vi "GeoData.vi"() -> ()   [LabVIEW 2017] (continued)
H1\n70391\t22007\tPaincourtville\tLA\tAssumption Parish\tH1\n70301\t22007\tThibodaux\tLA\tAssumption Parish\tH1\n70339\t22007\tPierre part\tLA\tAssumption Parish\tH1\n71362\t22009\tPlaucheville\tLA\tAvoyelles Parish\tH1\n71360\t22009\tPineville\tLA\tAvoyelles Parish\tH1\n71331\t22009\tEffie\tLA\tAvoyelles Parish\tH1\n71339\t22009\tHamburg\tLA\tAvoyelles Parish\tH1\n71350\t22009\tMansura\tLA\tAvoyelles Parish\tH1\n71353\t22009\tMelville\tLA\tAvoyelles Parish\tH1\n71355\t22009\tMoreauville\tLA\tAvoyelles Parish\tH1\n71328\t22009\tDeville\tLA\tAvoyelles Parish\tH1\n71323\t22009\tCenter point\tLA\tAvoyelles Parish\tH1\n71367\t22009\tSaint landry\tLA\tAvoyelles Parish\tH1\n71322\t22009\tBunkie\tLA\tAvoyelles Parish\tH1\n71327\t22009\tCottonport\tLA\tAvoyelles Parish\tH1\n71320\t22009\tBordelonville\tLA\tAvoyelles Parish\tH1\n71369\t22009\tSimmesport\tLA\tAvoyelles Parish\tH1\n71329\t22009\tDupont\tLA\tAvoyelles Parish\tH1\n71351\t22009\tMarksville\tLA\tAvoyelles Parish\tH1\n71341\t22009\tHessmer\tLA\tAvoyelles Parish\tH1\n71356\t22009\tMorrow\tLA\tAvoyelles Parish\tH1\n71333\t22009\tEvergreen\tLA\tAvoyelles Parish\tH1\n70653\t22011\tMerryville\tLA\tBeauregard Parish\tH1\n70662\t22011\tSugartown\tLA\tBeauregard Parish\tH1\n70633\t22011\tDequincy\tLA\tBeauregard Parish\tH1\n70637\t22011\tDry creek\tLA\tBeauregard Parish\tH1\n70634\t22011\tDeridder\tLA\tBeauregard Parish\tH1\n70657\t22011\tRagley\tLA\tBeauregard Parish\tH1\n70660\t22011\tSinger\tLA\tBeauregard Parish\tH1\n70652\t22011\tLongville\tLA\tBeauregard Parish\tH1\n70661\t22011\tStarks\tLA\tBeauregard Parish\tH1\n71070\t22013\tSaline\tLA\tBienville Parish\tH1\n71008\t22013\tBienville\tLA\tBienville Parish\tH1\n71275\t22013\tSimsboro\tLA\tBienville Parish\tH1\n71016\t22013\tCastor\tLA\tBienville Parish\tH1\n71024\t22013\tDubberly\tLA\tBienville Parish\tH1\n71055\t22013\tMinden\tLA\tBienville Parish\tH1\n71028\t22013\tGibsland\tLA\tBienville Parish\tH1\n71045\t22013\tJamestown\tLA\tBienville Parish\tH1\n71268\t22013\tQuitman\tLA\tBienville Parish\tH1\n71039\t22013\tHeflin\tLA\tBienville Parish\tH1\n71001\t22013\tArcadia\tLA\tBienville Parish\tH1\n71068\t22013\tRinggold\tLA\tBienville Parish\tH1\n71251\t22013\tJonesboro\tLA\tBienville Parish\tH1\n71080\t22013\tTaylor\tLA\tBienville Parish\tH1\n71006\t22015\tBenton\tLA\tBossier Parish\tH1\n71075\t22015\tSpringhill\tLA\tBossier Parish\tH1\n71067\t22015\tPrinceton\tLA\tBossier Parish\tH1\n71171\t22015\tBossier city\tLA\tBossier Parish\tH1\n71071\t22015\tSarepta\tLA\tBossier Parish\tH1\n71110\t22015\tBarksdale afb\tLA\tBossier Parish\tH1\n71111\t22015\tBossier city\tLA\tBossier Parish\tH1\n71105\t22015\tShreveport\tLA\tBossier Parish\tH1\n71113\t22015\tBossier city\tLA\tBossier Parish\tH1\n71106\t22015\tShreveport\tLA\tBossier Parish\tH1\n71104\t22015\tShreveport\tLA\tBossier Parish\tH1\n71101\t22015\tShreveport\tLA\tBossier Parish\tH1\n71137\t22015\tShreveport\tLA\tBossier Parish\tH1\n71112\t22015\tBossier city\tLA\tBossier Parish\tH1\n71172\t22015\tBossier city\tLA\tBossier Parish\tH1\n71064\t22015\tPlain dealing\tLA\tBossier Parish\tH1\n71115\t22015\tShreveport\tLA\tBossier Parish\tH1\n71051\t22015\tElm grove\tLA\tBossier Parish\tH1\n71037\t22015\tHaughton\tLA\tBossier Parish\tH1\n71023\t22015\tDoyline\tLA\tBossier Parish\tH1\n71107\t22015\tShreveport\tLA\tBossier Parish\tH1\n71018\t22015\tCotton valley\tLA\tBossier Parish\tH1\n71103\t22017\tShreveport\tLA\tCaddo Parish\tH1\n71004\t22017\tBelcher\tLA\tCaddo Parish\tH1\n71047\t22017\tKeithville\tLA\tCaddo Parish\tH1\n71046\t22017\tKeatchie\tLA\tCaddo Parish\tH1\n71044\t22017\tIda\tLA\tCaddo Parish\tH1\n71105\t22017\tShreveport\tLA\tCaddo Parish\tH1\n71134\t22017\tShreveport\tLA\tCaddo Parish\tH1\n71148\t22017\tShreveport\tLA\tCaddo Parish\tH1\n71029\t22017\tGilliam\tLA\tCaddo Parish\tH1\n71009\t22017\tBlanchard\tLA\tCaddo Parish\tH1\n71106\t22017\tShreveport\tLA\tCaddo Parish\tH1\n71104\t22017\tShreveport\tLA\tCaddo Parish\tH1\n71101\t22017\tShreveport\tLA\tCaddo Parish\tH1\n71061\t22017\tOil city\tLA\tCaddo Parish\tH1\n71136\t22017\tShreveport\tLA\tCaddo Parish\tH1\n71163\t22017\tShreveport\tLA\tCaddo Parish\tH1\n71109\t22017\tShreveport\tLA\tCaddo Parish\tH1\n71118\t22017\tShreveport\tLA\tCaddo Parish\tH1\n71119\t22017\tShreveport\tLA\tCaddo Parish\tH1\n71133\t22017\tShreveport\tLA\tCaddo Parish\tH1\n71033\t22017\tGreenwood\tLA\tCaddo Parish\tH1\n71060\t22017\tMooringsport\tLA\tCaddo Parish\tH1\n71069\t22017\tRodessa\tLA\tCaddo Parish\tH1\n71149\t22017\tShreveport\tLA\tCaddo Parish\tH1\n71162\t22017\tShreveport\tLA\tCaddo Parish\tH1\n71115\t22017\tShreveport\tLA\tCaddo Parish\tH1\n71043\t22017\tHosston\tLA\tCaddo Parish\tH1\n71165\t22017\tShreveport\tLA\tCaddo Parish\tH1\n71166\t22017\tShreveport\tLA\tCaddo Parish\tH1\n71129\t22017\tShreveport\tLA\tCaddo Parish\tH1\n71082\t22017\tVivian\tLA\tCaddo Parish\tH1\n71108\t22017\tShreveport\tLA\tCaddo Parish\tH1\n71138\t22017\tShreveport\tLA\tCaddo Parish\tH1\n71107\t22017\tShreveport\tLA\tCaddo Parish\tH1\n71135\t22017\tShreveport\tLA\tCaddo Parish\tH1\n71007\t22017\tBethany\tLA\tCaddo Parish\tH1\n71164\t22017\tShreveport\tLA\tCaddo Parish\tH1\n71161\t22017\tShreveport\tLA\tCaddo Parish\tH1\n71102\t22017\tShreveport\tLA\tCaddo Parish\tH1\n70605\t22019\tLake charles\tLA\tCalcasieu Parish\tH1\n70665\t22019\tSulphur\tLA\tCalcasieu Parish\tH1\n70601\t22019\tLake charles\tLA\tCalcasieu Parish\tH1\n70630\t22019\tBell city\tLA\tCalcasieu Parish\tH1\n70606\t22019\tLake charles\tLA\tCalcasieu Parish\tH1\n70633\t22019\tDequincy\tLA\tCalcasieu Parish\tH1\n70663\t22019\tSulphur\tLA\tCalcasieu Parish\tH1\n70612\t22019\tLake charles\tLA\tCalcasieu Parish\tH1\n70607\t22019\tLake charles\tLA\tCalcasieu Parish\tH1\n70629\t22019\tLake charles\tLA\tCalcasieu Parish\tH1\n70602\t22019\tLake charles\tLA\tCalcasieu Parish\tH1\n70647\t22019\tIowa\tLA\tCalcasieu Parish\tH1\n70657\t22019\tRagley\tLA\tCalcasieu Parish\tH1\n70646\t22019\tHayes\tLA\tCalcasieu Parish\tH1\n70611\t22019\tLake charles\tLA\tCalcasieu Parish\tH1\n70615\t22019\tLake charles\tLA\tCalcasieu Parish\tH1\n70669\t22019\tWestlake\tLA\tCalcasieu Parish\tH1\n70668\t22019\tVinton\tLA\tCalcasieu Parish\tH1\n70661\t22019\tStarks\tLA\tCalcasieu Parish\tH1\n70616\t22019\tLake charles\tLA\tCalcasieu Parish\tH1\n71465\t22021\tOlla\tLA\tCaldwell Parish\tH1\n71435\t22021\tGrayson\tLA\tCaldwell Parish\tH1\n71418\t22021\tColumbia\tLA\tCaldwell Parish\tH1\n71441\t22021\tKelly\tLA\tCaldwell Parish\tH1\n71415\t22021\tClarks\tLA\tCaldwell Parish\tH1\n70630\t22023\tBell city\tLA\tCameron Parish\tH1\n70542\t22023\tGueydan\tLA\tCameron Parish\tH1\n70645\t22023\tHackberry\tLA\tCameron Parish\tH1\n70606\t22023\tLake charles\tLA\tCameron Parish\tH1\n70643\t22023\tGrand chenier\tLA\tCameron Parish\tH1\n70607\t22023\tLake charles\tLA\tCameron Parish\tH1\n70631\t22023\tCameron\tLA\tCameron Parish\tH1\n70549\t22023\tLake arthur\tLA\tCameron Parish\tH1\n70632\t22023\tCreole\tLA\tCameron Parish\tH1\n71340\t22025\tHarrisonburg\tLA\tCatahoula Parish\tH1\n71363\t22025\tRhinehart\tLA\tCatahoula Parish\tH1\n71368\t22025\tSicily island\tLA\tCatahoula Parish\tH1\n71465\t22025\tOlla\tLA\tCatahoula Parish\tH1\n71354\t22025\tMonterey\tLA\tCatahoula Parish\tH1\n71401\t22025\tAimwell\tLA\tCatahoula Parish\tH1\n71418\t22025\tColumbia\tLA\tCatahoula Parish\tH1\n71425\t22025\tEnterprise\tLA\tCatahoula Parish\tH1\n71343\t22025\tJonesville\tLA\tCatahoula Parish\tH1\n71326\t22025\tClayton\tLA\tCatahoula Parish\tH1\n71256\t22027\tLillie\tLA\tClaiborne Parish\tH1\n71038\t22027\tHaynesville\tLA\tClaiborne Parish\tH1\n71048\t22027\tLisbon\tLA\tClaiborne Parish\tH1\n71222\t22027\tBernice\tLA\tClaiborne Parish\tH1\n71003\t22027\tAthens\tLA\tClaiborne Parish\tH1\n71055\t22027\tMinden\tLA\tClaiborne Parish\tH1\n71028\t22027\tGibsland\tLA\tClaiborne Parish\tH1\n71235\t22027\tDubach\tLA\tClaiborne Parish\tH1\n71001\t22027\tArcadia\tLA\tClaiborne Parish\tH1\n71040\t22027\tHomer\tLA\tClaiborne Parish\tH1\n71079\t22027\tSummerfield\tLA\tClaiborne Parish\tH1\n71373\t22029\tVidalia\tLA\tConcordia Parish\tH1\n71316\t22029\tAcme\tLA\tConcordia Parish\tH1\n71354\t22029\tMonterey\tLA\tConcordia Parish\tH1\n71334\t22029\tFerriday\tLA\tConcordia Parish\tH1\n71343\t22029\tJonesville\tLA\tConcordia Parish\tH1\n71326\t22029\tClayton\tLA\tConcordia Parish\tH1\n71063\t22031\tPelican\tLA\tDe Soto Parish\tH1\n71046\t22031\tKeatchie\tLA\tDe Soto Parish\tH1\n71030\t22031\tGloster\tLA\tDe Soto Parish\tH1\n71049\t22031\tLogansport\tLA\tDe Soto Parish\tH1\n71052\t22031\tMansfield\tLA\tDe Soto Parish\tH1\n71032\t22031\tGrand cane\tLA\tDe Soto Parish\tH1\n71078\t22031\tStonewall\tLA\tDe Soto Parish\tH1\n71419\t22031\tConverse\tLA\tDe Soto Parish\tH1\n71027\t22031\tFrierson\tLA\tDe Soto Parish\tH1\n70805\t22033\tBaton rouge\tLA\tEast Baton Rouge Parish\tH1\n70815\t22033\tBaton rouge\tLA\tEast Baton Rouge Parish\tH1\n70770\t22033\tPride\tLA\tEast Baton Rouge Parish\tH1\n70802\t22033\tBaton rouge\tLA\tEast Baton Rouge Parish\tH1\n70814\t22033\tBaton rouge\tLA\tEast Baton Rouge Parish\tH1\n70817\t22033\tBaton rouge\tLA\tEast Baton Rouge Parish\tH1\n70898\t22033\tBaton rouge\tLA\tEast Baton Rouge Parish\tH1\n70819\t22033\tBaton rouge\tLA\tEast Baton Rouge Parish\tH1\n70827\t22033\tBaton rouge\tLA\tEast Baton Rouge Parish\tH1\n70810\t22033\tBaton rouge\tLA\tEast Baton Rouge Parish\tH1\n70748\t22033\tJackson\tLA\tEast Baton Rouge Parish\tH1\n70812\t22033\tBaton rouge\tLA\tEast Baton Rouge Parish\tH1\n70835\t22033\tBaton rouge\tLA\tEast Baton Rouge Parish\tH1\n70879\t22033\tBaton rouge\tLA\tEast Baton Rouge Parish\tH1\n70777\t22033\tSlaughter\tLA\tEast Baton Rouge Parish\tH1\n70807\t22033\tBaton rouge\tLA\tEast Baton Rouge Parish\tH1\n70739\t22033\tGreenwell springs\tLA\tEast Baton Rouge Parish\tH1\n70804\t22033\tBaton rouge\tLA\tEast Baton Rouge Parish\tH1\n70874\t22033\tBaton rouge\tLA\tEast Baton Rouge Parish\tH1\n70896\t22033\tBaton rouge\tLA\tEast Baton Rouge Parish\tH1\n70722\t22033\tClinton\tLA\tEast Baton Rouge Parish\tH1\n70806\t22033\tBaton rouge\tLA\tEast Baton Rouge Parish\tH1\n70808\t22033\tBaton rouge\tLA\tEast Baton Rouge Parish\tH1\n70821\t22033\tBaton rouge\tLA\tEast Baton Rouge Parish\tH1\n70714\t22033\tBaker\tLA\tEast Baton Rouge Parish\tH1\n70818\t22033\tBaton rouge\tLA\tEast Baton Rouge Parish\tH1\n70836\t22033\tBaton rouge\tLA\tEast Baton Rouge Parish\tH1\n70892\t22033\tBaton rouge\tLA\tEast Baton Rouge Parish\tH1\n70884\t22033\tBaton rouge\tLA\tEast Baton Rouge Parish\tH1\n70893\t22033\tBaton rouge\tLA\tEast Baton Rouge Parish\tH1\n70809\t22033\tBaton rouge\tLA\tEast Baton Rouge Parish\tH1\n70801\t22033\tBaton rouge\tLA\tEast Baton Rouge Parish\tH1\n70791\t22033\tZachary\tLA\tEast Baton Rouge Parish\tH1\n70811\t22033\tBaton rouge\tLA\tEast Baton Rouge Parish\tH1\n70767\t22033\tPort allen\tLA\tEast Baton Rouge Parish\tH1\n70816\t22033\tBaton rouge\tLA\tEast Baton Rouge Parish\tH1\n70820\t22033\tBaton rouge\tLA\tEast Baton Rouge Parish\tH1\n70825\t22033\tBaton rouge\tLA\tEast Baton Rouge Parish\tH1\n70895\t22033\tBaton rouge\tLA\tEast Baton Rouge Parish\tH1\n70704\t22033\tBaker\tLA\tEast Baton Rouge Parish\tH1\n70803\t22033\tBaton rouge\tLA\tEast Baton Rouge Parish\tH1\n71254\t22035\tLake providence\tLA\tEast Carroll Parish\tH1\n71286\t22035\tTransylvania\tLA\tEast Carroll Parish\tH1\n71276\t22035\tSondheimer\tLA\tEast Carroll Parish\tH1\n71237\t22035\tEpps\tLA\tEast Carroll Parish\tH1\n70748\t22037\tJackson\tLA\tEast Feliciana Parish\tH1\n70761\t22037\tNorwood\tLA\tEast Feliciana Parish\tH1\n70777\t22037\tSlaughter\tLA\tEast Feliciana Parish\tH1\n70722\t22037\tClinton\tLA\tEast Feliciana Parish\tH1\n70730\t22037\tEthel\tLA\tEast Feliciana Parish\tH1\n70791\t22037\tZachary\tLA\tEast Feliciana Parish\tH1\n70789\t22037\tWilson\tLA\tEast Feliciana Parish\tH1\n70580\t22039\tReddell\tLA\tEvangeline Parish\tH1\n70585\t22039\tTurkey creek\tLA\tEvangeline Parish\tH1\n70524\t22039\tChataignier\tLA\tEvangeline Parish\tH1\n70576\t22039\tPine prairie\tLA\tEvangeline Parish\tH1\n70586\t22039\tVille platte\tLA\tEvangeline Parish\tH1\n70589\t22039\tWashington\tLA\tEvangeline Parish\tH1\n71367\t22039\tSaint landry\tLA\tEvangeline Parish\tH1\n70554\t22039\tMamou\tLA\tEvangeline Parish\tH1\n70535\t22039\tEunice\tLA\tEvangeline Parish\tH1\n70515\t22039\tBasile\tLA\tEvangeline Parish\tH1\n71463\t22039\tOakdale\tLA\tEvangeline Parish\tH1\n71433\t22039\tGlenmora\tLA\tEvangeline Parish\tH1\n71325\t22039\tCheneyville\tLA\tEvangeline Parish\tH1\n70570\t22039\tOpelousas\tLA\tEvangeline Parish\tH1\n71269\t22041\tRayville\tLA\tFranklin Parish\tH1\n71368\t22041\tSicily island\tLA\tFranklin Parish\tH1\n71219\t22041\tBaskin\tLA\tFranklin Parish\tH1\n71243\t22041\tFort necessity\tLA\tFranklin Parish\tH1\n71295\t22041\tWinnsboro\tLA\tFranklin Parish\tH1\n71249\t22041\tJigger\tLA\tFranklin Parish\tH1\n71336\t22041\tGilbert\tLA\tFranklin Parish\tH1\n71378\t22041\tWisner\tLA\tFranklin Parish\tH1\n71230\t22041\tCrowville\tLA\tFranklin Parish\tH1\n71232\t22041\tDelhi\tLA\tFranklin Parish\tH1\n71324\t22041\tChase\tLA\tFranklin Parish\tH1\n71360\t22043\tPineville\tLA\tGrant Parish\tH1\n71407\t22043\tBentley\tLA\tGrant Parish\tH1\n71423\t22043\tDry prong\tLA\tGrant Parish\tH1\n71404\t22043\tAtlanta\tLA\tGrant Parish\tH1\n71454\t22043\tMontgomery\tLA\tGrant Parish\tH1\n71417\t22043\tColfax\tLA\tGrant Parish\tH1\n71432\t22043\tGeorgetown\tLA\tGrant Parish\tH1\n71467\t22043\tPollock\tLA\tGrant Parish\tH1\n70560\t22045\tNew iberia\tLA\tIberia Parish\tH1\n70592\t22045\tYoungsville\tLA\tIberia Parish\tH1\n70513\t22045\tAvery island\tLA\tIberia Parish\tH1\n70563\t22045\tNew iberia\tLA\tIberia Parish\tH1\n70569\t22045\tLydia\tLA\tIberia Parish\tH1\n70544\t22045\tJeanerette\tLA\tIberia Parish\tH1\n70533\t22045\tErath\tLA\tIberia Parish\tH1\n70528\t22045\tDelcambre\tLA\tIberia Parish\tH1\n70582\t22045\tSaint martinville\tLA\tIberia Parish\tH1\n70552\t22045\tLoreauville\tLA\tIberia Parish\tH1\n70562\t22045\tNew iberia\tLA\tIberia Parish\tH1\n70518\t22045\tBroussard\tLA\tIberia Parish\tH1\n70346\t22047\tDonaldsonville\tLA\tIberville Parish\tH1\n70764\t22047\tPlaquemine\tLA\tIberville Parish\tH1\n70740\t22047\tGrosse tete\tLA\tIberville Parish\tH1\n70721\t22047\tCarville\tLA\tIberville Parish\tH1\n70772\t22047\tRosedale\tLA\tIberville Parish\tH1\n70776\t22047\tSaint gabriel\tLA\tIberville Parish\tH1\n70757\t22047\tMaringouin\tLA\tIberville Parish\tH1\n70780\t22047\tSunshine\tLA\tIberville Parish\tH1\n70788\t22047\tWhite castle\tLA\tIberville Parish\tH1\n71238\t22049\tEros\tLA\tJackson Parish\tH1\n71435\t22049\tGrayson\tLA\tJackson Parish\tH1\n71225\t22049\tCalhoun\tLA\tJackson Parish\tH1\n71247\t22049\tHodge\tLA\tJackson Parish\tH1\n71268\t22049\tQuitman\tLA\tJackson Parish\tH1\n71226\t22049\tChatham\tLA\tJackson Parish\tH1\n71251\t22049\tJonesboro\tLA\tJackson Parish\tH1\n71227\t22049\tChoudrant\tLA\tJackson Parish\tH1\n71270\t22049\tRuston\tLA\tJackson Parish\tH1\n70058\t22051\tHarvey\tLA\tJefferson Parish\tH1\n70094\t22051\tWestwego\tLA\tJefferson Parish\tH1\n70064\t22051\tKenner\tLA\tJefferson Parish\tH1\n70073\t22051\tMarrero\tLA\tJefferson Parish\tH1\n70121\t22051\tNew orleans\tLA\tJefferson Parish\tH1\n70063\t22051\tKenner\tLA\tJefferson Parish\tH1\n70181\t22051\tNew orleans\tLA\tJefferson Parish\tH1\n70010\t22051\tMetairie\tLA\tJefferson Parish\tH1\n70003\t22051\tMetairie\tLA\tJefferson Parish\tH1\n70115\t22051\tNew orleans\tLA\tJefferson Parish\tH1\n70183\t22051\tNew orleans\tLA\tJefferson Parish\tH1\n70009\t22051\tMetairie\tLA\tJefferson Parish\tH1\n70055\t22051\tMetairie\tLA\tJefferson Parish\tH1\n70065\t22051\tKenner\tLA\tJefferson Parish\tH1\n70062\t22051\tKenner\tLA\tJefferson Parish\tH1\n70123\t22051\tNew orleans\tLA\tJefferson Parish\tH1\n70011\t22051\tMetairie\tLA\tJefferson Parish\tH1\n70005\t22051\tMetairie\tLA\tJefferson Parish\tH1\n70033\t22051\tMetairie\tLA\tJefferson Parish\tH1\n70031\t22051\tAma\tLA\tJefferson Parish\tH1\n70002\t22051\tMetairie\tLA\tJefferson Parish\tH1\n70053\t22051\tGretna\tLA\tJefferson Parish\tH1\n70067\t22051\tLafitte\tLA\tJefferson Parish\tH1\n70059\t22051\tHarvey\tLA\tJefferson Parish\tH1\n70006\t22051\tMetairie\tLA\tJefferson Parish\tH1\n70036\t22051\tBarataria\tLA\tJefferson Parish\tH1\n70004\t22051\tMetairie\tLA\tJefferson Parish\tH1\n70056\t22051\tGretna\tLA\tJefferson Parish\tH1\n70114\t22051\tNew orleans\tLA\tJefferson Parish\tH1\n70001\t22051\tMetairie\tLA\tJefferson Parish\tH1\n70054\t22051\tGretna\tLA\tJefferson Parish\tH1\n70072\t22051\tMarrero\tLA\tJefferson Parish\tH1\n70358\t22051\tGrand isle\tLA\tJefferson Parish\tH1\n70096\t22051\tWestwego\tLA\tJefferson Parish\tH1\n70591\t22053\tWelsh\tLA\tJefferson Davis Parish\tH1\n70640\t22053\tFenton\tLA\tJefferson Davis Parish\tH1\n70546\t22053\tJennings\tLA\tJefferson Davis Parish\tH1\n70650\t22053\tLacassine\tLA\tJefferson Davis Parish\tH1\n70549\t22053\tLake arthur\tLA\tJefferson Davis Parish\tH1\n70647\t22053\tIowa\tLA\tJefferson Davis Parish\tH1\n70532\t22053\tElton\tLA\tJefferson Davis Parish\tH1\n70657\t22053\tRagley\tLA\tJefferson Davis Parish\tH1\n70611\t22053\tLake charles\tLA\tJefferson Davis Parish\tH1\n70648\t22053\tKinder\tLA\tJefferson Davis Parish\tH1\n70581\t22053\tRoanoke\tLA\tJefferson Davis Parish\tH1\n70517\t22055\tBreaux bridge\tLA\tLafayette Parish\tH1\n70560\t22055\tNew iberia\tLA\tLafayette Parish\tH1\n70501\t22055\tLafayette\tLA\tLafayette Parish\tH1\n70506\t22055\tLafayette\tLA\tLafayette Parish\tH1\n70592\t22055\tYoungsville\tLA\tLafayette Parish\tH1\n70502\t22055\tLafayette\tLA\tLafayette Parish\tH1\n70503\t22055\tLafayette\tLA\tLafayette Parish\tH1\n70525\t22055\tChurch point\tLA\tLafayette Parish\tH1\n70558\t22055\tMilton\tLA\tLafayette Parish\tH1\n70507\t22055\tLafayette\tLA\tLafayette Parish\tH1\n70555\t22055\tMaurice\tLA\tLafayette Parish\tH1\n70508\t22055\tLafayette\tLA\tLafayette Parish\tH1\n70505\t22055\tLafayette\tLA\tLafayette Parish\tH1\n70578\t22055\tRayne\tLA\tLafayette Parish\tH1\n70529\t22055\tDuson\tLA\tLafayette Parish\tH1\n70504\t22055\tLafayette\tLA\tLafayette Parish\tH1\n70518\t22055\tBroussard\tLA\tLafayette Parish\tH1\n70520\t22055\tCarencro\tLA\tLafayette Parish\tH1\n70583\t22055\tScott\tLA\tLafayette Parish\tH1\n70596\t22055\tLafayette\tLA\tLafayette Parish\tH1\n70509\t22055\tLafayette\tLA\tLafayette Parish\tH1\n70598\t22055\tLafayette\tLA\tLafayette Parish\tH1\n70374\t22057\tLockport\tLA\tLafourche Parish\tH1\n70357\t22057\tGolden meadow\tLA\tLafourche Parish\tH1\n70343\t22057\tBourg\tLA\tLafourche Parish\tH1\n70354\t22057\tGalliano\tLA\tLafourche Parish\tH1\n70364\t22057\tHouma\tLA\tLafourche Parish\tH1\n70345\t22057\tCut off\tLA\tLafourche Parish\tH1\n70394\t22057\tRaceland\tLA\tLafourche Parish\tH1\n70355\t22057\tGheens\tLA\tLafourche Parish\tH1\n70359\t22057\tGray\tLA\tLafourche Parish\tH1\n70371\t22057\tKraemer\tLA\tLafourche Parish\tH1\n70301\t22057\tThibodaux\tLA\tLafourche Parish\tH1\n70375\t22057\tMathews\tLA\tLafourche Parish\tH1\n70030\t22057\tDes allemands\tLA\tLafourche Parish\tH1\n70377\t22057\tMontegut\tLA\tLafourche Parish\tH1\n70373\t22057\tLarose\tLA\tLafourche Parish\tH1\n71479\t22059\tTullos\tLA\tLa Salle Parish\tH1\n71465\t22059\tOlla\tLA\tLa Salle Parish\tH1\n71435\t22059\tGrayson\tLA\tLa Salle Parish\tH1\n71480\t22059\tUrania\tLA\tLa Salle Parish\tH1\n71441\t22059\tKelly\tLA\tLa Salle Parish\tH1\n71342\t22059\tJena\tLA\tLa Salle Parish\tH1\n71343\t22059\tJonesville\tLA\tLa Salle Parish\tH1\n71371\t22059\tTrout\tLA\tLa Salle Parish\tH1\n71275\t22061\tSimsboro\tLA\tLincoln Parish\tH1\n71272\t22061\tRuston\tLA\tLincoln Parish\tH1\n71234\t22061\tDownsville\tLA\tLincoln Parish\tH1\n71003\t22061\tAthens\tLA\tLincoln Parish\tH1\n71273\t22061\tRuston\tLA\tLincoln Parish\tH1\n71241\t22061\tFarmerville\tLA\tLincoln Parish\tH1\n71235\t22061\tDubach\tLA\tLincoln Parish\tH1\n71001\t22061\tArcadia\tLA\tLincoln Parish\tH1\n71227\t22061\tChoudrant\tLA\tLincoln Parish\tH1\n71245\t22061\tGrambling\tLA\tLincoln Parish\tH1\n71270\t22061\tRuston\tLA\tLincoln Parish\tH1\n70706\t22063\tDenham springs\tLA\tLivingston Parish\tH1\n70403\t22063\tHammond\tLA\tLivingston Parish\tH1\n70466\t22063\tTickfaw\tLA\tLivingston Parish\tH1\n70754\t22063\tLivingston\tLA\tLivingston Parish\tH1\n70774\t22063\tSaint amant\tLA\tLivingston Parish\tH1\n70727\t22063\tDenham springs\tLA\tLivingston Parish\tH1\n70726\t22063\tDenham springs\tLA\tLivingston Parish\tH1\n70711\t22063\tAlbany\tLA\tLivingston Parish\tH1\n70786\t22063\tWatson\tLA\tLivingston Parish\tH1\n70462\t22063\tSpringfield\tLA\tLivingston Parish\tH1\n70453\t22063\tPine grove\tLA\tLivingston Parish\tH1\n70449\t22063\tMaurepas\tLA\tLivingston Parish\tH1\n70422\t22063\tAmite\tLA\tLivingston Parish\tH1\n70443\t22063\tIndependence\tLA\tLivingston Parish\tH1\n70785\t22063\tWalker\tLA\tLivingston Parish\tH1\n70744\t22063\tHolden\tLA\tLivingston Parish\tH1\n70733\t22063\tFrench settlement\tLA\tLivingston Parish\tH1\n71233\t22065\tDelta\tLA\tMadison Parish\tH1\n71237\t22065\tEpps\tLA\tMadison Parish\tH1\n71232\t22065\tDelhi\tLA\tMadison Parish\tH1\n71282\t22065\tTallulah\tLA\tMadison Parish\tH1\n71280\t22067\tSterlington\tLA\tMorehouse Parish\tH1\n71261\t22067\tMer rouge\tLA\tMorehouse Parish\tH1\n71269\t22067\tRayville\tLA\tMorehouse Parish\tH1\n71223\t22067\tBonita\tLA\tMorehouse Parish\tH1\n71264\t22067\tOak ridge\tLA\tMorehouse Parish\tH1\n71229\t22067\tCollinston\tLA\tMorehouse Parish\tH1\n71250\t22067\tJones\tLA\tMorehouse Parish\tH1\n71220\t22067\tBastrop\tLA\tMorehouse Parish\tH1\n71070\t22069\tSaline\tLA\tNatchitoches Parish\tH1\n71063\t22069\tPelican\tLA\tNatchitoches Parish\tH1\n71416\t22069\tCloutierville\tLA\tNatchitoches Parish\tH1\n71468\t22069\tProvencal\tLA\tNatchitoches Parish\tH1\n71414\t22069\tClarence\tLA\tNatchitoches Parish\tH1\n71447\t22069\tLena\tLA\tNatchitoches Parish\tH1\n71456\t22069\tNatchez\tLA\tNatchitoches Parish\tH1\n71066\t22069\tPowhatan\tLA\tNatchitoches Parish\tH1\n71457\t22069\tNatchitoches\tLA\tNatchitoches Parish\tH1\n71455\t22069\tMora\tLA\tNatchitoches Parish\tH1\n71031\t22069\tGoldonna\tLA\tNatchitoches Parish\tH1\n71497\t22069\tNatchitoches\tLA\tNatchitoches Parish\tH1\n71016\t22069\tCastor\tLA\tNatchitoches Parish\tH1\n71002\t22069\tAshland\tLA\tNatchitoches Parish\tH1\n71411\t22069\tCampti\tLA\tNatchitoches Parish\tH1\n71452\t22069\tMelrose\tLA\tNatchitoches Parish\tH1\n71065\t22069\tPleasant hill\tLA\tNatchitoches Parish\tH1\n71427\t22069\tFlatwoods\tLA\tNatchitoches Parish\tH1\n71019\t22069\tCoushatta\tLA\tNatchitoches Parish\tH1\n71458\t22069\tNatchitoches\tLA\tNatchitoches Parish\tH1\n71428\t22069\tFlora\tLA\tNatchitoches Parish\tH1\n71434\t22069\tGorum\tLA\tNatchitoches Parish\tH1\n71469\t22069\tRobeline\tLA\tNatchitoches Parish\tH1\n71450\t22069\tMarthaville\tLA\tNatchitoches Parish\tH1\n70121\t22071\tNew orleans\tLA\tOrleans Parish\tH6\n70130\t22071\tNew orleans\tLA\tOrleans Parish\tH6\n70182\t22071\tNew orleans\tLA\tOrleans Parish\tH6\n70148\t22071\tNew orleans\tLA\tOrleans Parish\tH6\n70145\t22071\tNew orleans\tLA\tOrleans Parish\tH6\n70129\t22071\tNew orleans\tLA\tOrleans Parish\tH6\n70112\t22071\tNew orleans\tLA\tOrleans Parish\tH6\n70115\t22071\tNew orleans\tLA\tOrleans Parish\tH6\n70117\t22071\tNew orleans\tLA\tOrleans Parish\tH6\n70125\t22071\tNew orleans\tLA\tOrleans Parish\tH6\n70177\t22071\tNew orleans\tLA\tOrleans Parish\tH6\n70157\t22071\tNew orleans\tLA\tOrleans Parish\tH6\n70141\t22071\tNew orleans\tLA\tOrleans Parish\tH6\n70127\t22071\tNew orleans\tLA\tOrleans Parish\tH6\n70118\t22071\tNew orleans\tLA\tOrleans Parish\tH6\n70116\t22071\tNew orleans\tLA\tOrleans Parish\tH6\n70152\t22071\tNew orleans\tLA\tOrleans Parish\tH6\n70158\t22071\tNew orleans\tLA\tOrleans Parish\tH6\n70175\t22071\tNew orleans\tLA\tOrleans Parish\tH6\n70184\t22071\tNew orleans\tLA\tOrleans Parish\tH6\n70128\t22071\tNew orleans\tLA\tOrleans Parish\tH6\n70178\t22071\tNew orleans\tLA\tOrleans Parish\tH6\n70163\t22071\tNew orleans\tLA\tOrleans Parish\tH6\n70174\t22071\tNew orleans\tLA\tOrleans Parish\tH6\n70139\t22071\tNew orleans\tLA\tOrleans Parish\tH6\n70150\t22071\tNew orleans\tLA\tOrleans Parish\tH6\n70146\t22071\tNew orleans\tLA\tOrleans Parish\tH6\n70119\t22071\tNew orleans\tLA\tOrleans Parish\tH6\n70122\t22071\tNew orleans\tLA\tOrleans Parish\tH6\n70126\t22071\tNew orleans\tLA\tOrleans Parish\tH6\n70131\t22071\tNew orleans\tLA\tOrleans Parish\tH6\n70151\t22071\tNew orleans\tLA\tOrleans Parish\tH6\n70172\t22071\tNew orleans\tLA\tOrleans Parish\tH6\n70185\t22071\tNew orleans\tLA\tOrleans Parish\tH6\n70190\t22071\tNew orleans\tLA\tOrleans Parish\tH6\n70170\t22071\tNew orleans\tLA\tOrleans Parish\tH6\n70186\t22071\tNew orleans\tLA\tOrleans Parish\tH6\n70176\t22071\tNew orleans\tLA\tOrleans Parish\tH6\n70165\t22071\tNew orleans\tLA\tOrleans Parish\tH6\n70124\t22071\tNew orleans\tLA\tOrleans Parish\tH6\n70114\t22071\tNew orleans\tLA\tOrleans Parish\tH6\n70113\t22071\tNew orleans\tLA\tOrleans Parish\tH6\n70156\t22071\tNew orleans\tLA\tOrleans Parish\tH6\n70179\t22071\tNew orleans\tLA\tOrleans Parish\tH6\n70153\t22071\tNew orleans\tLA\tOrleans Parish\tH6\n71202\t22073\tMonroe\tLA\tOuachita Parish\tH1\n71238\t22073\tEros\tLA\tOuachita Parish\tH1\n71207\t22073\tMonroe\tLA\tOuachita Parish\tH1\n71280\t22073\tSterlington\tLA\tOuachita Parish\tH1\n71418\t22073\tColumbia\tLA\tOuachita Parish\tH1\n71203\t22073\tMonroe\tLA\tOuachita Parish\tH1\n71229\t22073\tCollinston\tLA\tOuachita Parish\tH1\n71225\t22073\tCalhoun\tLA\tOuachita Parish\tH1\n71234\t22073\tDownsville\tLA\tOuachita Parish\tH1\n71292\t22073\tWest monroe\tLA\tOuachita Parish\tH1\n71209\t22073\tMonroe\tLA\tOuachita Parish\tH1\n71211\t22073\tMonroe\tLA\tOuachita Parish\tH1\n71201\t22073\tMonroe\tLA\tOuachita Parish\tH1\n71294\t22073\tWest monroe\tLA\tOuachita Parish\tH1\n71213\t22073\tMonroe\tLA\tOuachita Parish\tH1\n71281\t22073\tSwartz\tLA\tOuachita Parish\tH1\n71212\t22073\tMonroe\tLA\tOuachita Parish\tH1\n71210\t22073\tMonroe\tLA\tOuachita Parish\tH1\n71227\t22073\tChoudrant\tLA\tOuachita Parish\tH1\n71291\t22073\tWest monroe\tLA\tOuachita Parish\tH1\n71240\t22073\tFairbanks\tLA\tOuachita Parish\tH1\n70041\t22075\tBuras\tLA\tPlaquemines Parish\tH1\n70040\t22075\tBraithwaite\tLA\tPlaquemines Parish\tH1\n70093\t22075\tBelle chasse\tLA\tPlaquemines Parish\tH1\n70050\t22075\tEmpire\tLA\tPlaquemines Parish\tH1\n70091\t22075\tVenice\tLA\tPlaquemines Parish\tH1\n70083\t22075\tPort sulphur\tLA\tPlaquemines Parish\tH1\n70143\t22075\tNew orleans\tLA\tPlaquemines Parish\tH1\n70037\t22075\tBelle chasse\tLA\tPlaquemines Parish\tH1\n70082\t22075\tPointe a la hache\tLA\tPlaquemines Parish\tH1\n70749\t22077\tJarreau\tLA\tPointe Coupee Parish\tH1\n70752\t22077\tLakeland\tLA\tPointe Coupee Parish\tH1\n70773\t22077\tRougon\tLA\tPointe Coupee Parish\tH1\n70747\t22077\tInnis\tLA\tPointe Coupee Parish\tH1\n70715\t22077\tBatchelor\tLA\tPointe Coupee Parish\tH1\n70762\t22077\tOscar\tLA\tPointe Coupee Parish\tH1\n70755\t22077\tLivonia\tLA\tPointe Coupee Parish\tH1\n70736\t22077\tGlynn\tLA\tPointe Coupee Parish\tH1\n70756\t22077\tLottie\tLA\tPointe Coupee Parish\tH1\n70732\t22077\tFordoche\tLA\tPointe Coupee Parish\tH1\n70783\t22077\tVentress\tLA\tPointe Coupee Parish\tH1\n70757\t22077\tMaringouin\tLA\tPointe Coupee Parish\tH1\n70759\t22077\tMorganza\tLA\tPointe Coupee Parish\tH1\n70767\t22077\tPort allen\tLA\tPointe Coupee Parish\tH1\n70760\t22077\tNew roads\tLA\tPointe Coupee Parish\tH1\n70753\t22077\tLettsworth\tLA\tPointe Coupee Parish\tH1\n70729\t22077\tErwinville\tLA\tPointe Coupee Parish\tH1\n71438\t22079\tHineston\tLA\tRapides Parish\tH1\n71360\t22079\tPineville\tLA\tRapides Parish\tH1\n71430\t22079\tForest hill\tLA\tRapides Parish\tH1\n71447\t22079\tLena\tLA\tRapides Parish\tH1\n71330\t22079\tEcho\tLA\tRapides Parish\tH1\n71423\t22079\tDry prong\tLA\tRapides Parish\tH1\n71455\t22079\tMora\tLA\tRapides Parish\tH1\n71365\t22079\tRuby\tLA\tRapides Parish\tH1\n71302\t22079\tAlexandria\tLA\tRapides Parish\tH1\n71424\t22079\tElmer\tLA\tRapides Parish\tH1\n71485\t22079\tWoodworth\tLA\tRapides Parish\tH1\n71301\t22079\tAlexandria\tLA\tRapides Parish\tH1\n71328\t22079\tDeville\tLA\tRapides Parish\tH1\n71323\t22079\tCenter point\tLA\tRapides Parish\tH1\n71346\t22079\tLecompte\tLA\tRapides Parish\tH1\n71315\t22079\tAlexandria\tLA\tRapides Parish\tH1\n71409\t22079\tBoyce\tLA\tRapides Parish\tH1\n71472\t22079\tSieper\tLA\tRapides Parish\tH1\n71466\t22079\tOtis\tLA\tRapides Parish\tH1\n71477\t22079\tTioga\tLA\tRapides Parish\tH1\n71348\t22079\tLibuse\tLA\tRapides Parish\tH1\n71322\t22079\tBunkie\tLA\tRapides Parish\tH1\n71427\t22079\tFlatwoods\tLA\tRapides Parish\tH1\n71448\t22079\tLongleaf\tLA\tRapides Parish\tH1\n70656\t22079\tPitkin\tLA\tRapides Parish\tH1\n71405\t22079\tBall\tLA\tRapides Parish\tH1\n71463\t22079\tOakdale\tLA\tRapides Parish\tH1\n71307\t22079\tAlexandria\tLA\tRapides Parish\tH1\n71433\t22079\tGlenmora\tLA\tRapides Parish\tH1\n71467\t22079\tPollock\tLA\tRapides Parish\tH1\n71306\t22079\tAlexandria\tLA\tRapides Parish\tH1\n71325\t22079\tCheneyville\tLA\tRapides Parish\tH1\n71309\t22079\tAlexandria\tLA\tRapides Parish\tH1\n71359\t22079\tPineville\tLA\tRapides Parish\tH1\n71351\t22079\tMarksville\tLA\tRapides Parish\tH1\n71303\t22079\tAlexandria\tLA\tRapides Parish\tH1\n71115\t22081\tShreveport\tLA\tRed River Parish\tH1\n71052\t22081\tMansfield\tLA\tRed River Parish\tH1\n71068\t22081\tRinggold\tLA\tRed River Parish\tH1\n71019\t22081\tCoushatta\tLA\tRed River Parish\tH1\n71034\t22081\tHall summit\tLA\tRed River Parish\tH1\n71269\t22083\tRayville\tLA\tRichland Parish\tH1\n71418\t22083\tColumbia\tLA\tRichland Parish\tH1\n71264\t22083\tOak ridge\tLA\tRichland Parish\tH1\n71218\t22083\tArchibald\tLA\tRichland Parish\tH1\n71237\t22083\tEpps\tLA\tRichland Parish\tH1\n71279\t22083\tStart\tLA\tRichland Parish\tH1\n71259\t22083\tMangham\tLA\tRichland Parish\tH1\n71232\t22083\tDelhi\tLA\tRichland Parish\tH1\n71429\t22085\tFlorien\tLA\tSabine Parish\tH1\n71468\t22085\tProvencal\tLA\tSabine Parish\tH1\n71439\t22085\tHornbeck\tLA\tSabine Parish\tH1\n71406\t22085\tBelmont\tLA\tSabine Parish\tH1\n71462\t22085\tNoble\tLA\tSabine Parish\tH1\n71486\t22085\tZwolle\tLA\tSabine Parish\tH1\n71403\t22085\tAnacoco\tLA\tSabine Parish\tH1\n71065\t22085\tPleasant hill\tLA\tSabine Parish\tH1\n71419\t22085\tConverse\tLA\tSabine Parish\tH1\n71460\t22085\tNegreet\tLA\tSabine Parish\tH1\n71469\t22085\tRobeline\tLA\tSabine Parish\tH1\n71449\t22085\tMany\tLA\tSabine Parish\tH1\n71450\t22085\tMarthaville\tLA\tSabine Parish\tH1\n71426\t22085\tFisher\tLA\tSabine Parish\tH1\n70092\t22087\tViolet\tLA\tSt. Bernard Parish\tH1\n70032\t22087\tArabi\tLA\tSt. Bernard Parish\tH1\n70040\t22087\tBraithwaite\tLA\tSt. Bernard Parish\tH1\n70075\t22087\tMeraux\tLA\tSt. Bernard Parish\tH1\n70085\t22087\tSaint bernard\tLA\tSt. Bernard Parish\tH1\n70043\t22087\tChalmette\tLA\tSt. Bernard Parish\tH1\n70087\t22089\tSaint rose\tLA\tSt. Charles Parish\tH1\n70068\t22089\tLa place\tLA\tSt. Charles Parish\tH1\n70080\t22089\tParadis\tLA\tSt. Charles Parish\tH1\n70039\t22089\tBoutte\tLA\tSt. Charles Parish\tH1\n70031\t22089\tAma\tLA\tSt. Charles Parish\tH1\n70047\t22089\tDestrehan\tLA\tSt. Charles Parish\tH1\n70079\t22089\tNorco\tLA\tSt. Charles Parish\tH1\n70078\t22089\tNew sarpy\tLA\tSt. Charles Parish\tH1\n70057\t22089\tHahnville\tLA\tSt. Charles Parish\tH1\n70030\t22089\tDes allemands\tLA\tSt. Charles Parish\tH1\n70070\t22089\tLuling\tLA\tSt. Charles Parish\tH1\n70706\t22091\tDenham springs\tLA\tSt. Helena Parish\tH1\n70444\t22091\tKentwood\tLA\tSt. Helena Parish\tH1\n70453\t22091\tPine grove\tLA\tSt. Helena Parish\tH1\n70436\t22091\tFluker\tLA\tSt. Helena Parish\tH1\n70422\t22091\tAmite\tLA\tSt. Helena Parish\tH1\n70443\t22091\tIndependence\tLA\tSt. Helena Parish\tH1\n70441\t22091\tGreensburg\tLA\tSt. Helena Parish\tH1\n70744\t22091\tHolden\tLA\tSt. Helena Parish\tH1\n70346\t22093\tDonaldsonville\tLA\tSt. James Parish\tH1\n70792\t22093\tUncle sam\tLA\tSt. James Parish\tH1\n70086\t22093\tSaint james\tLA\tSt. James Parish\tH1\n70743\t22093\tHester\tLA\tSt. James Parish\tH1\n70723\t22093\tConvent\tLA\tSt. James Parish\tH1\n70090\t22093\tVacherie\tLA\tSt. James Parish\tH1\n70763\t22093\tPaulina\tLA\tSt. James Parish\tH1\n70052\t22093\tGramercy\tLA\tSt. James Parish\tH1\n70071\t22093\tLutcher\tLA\tSt. James Parish\tH1\n70084\t22095\tReserve\tLA\tSt. John the Baptist Parish\tH1\n70068\t22095\tLa place\tLA\tSt. John the Baptist Parish\tH1\n70076\t22095\tMount airy\tLA\tSt. John the Baptist Parish\tH1\n70090\t22095\tVacherie\tLA\tSt. John the Baptist Parish\tH1\n70069\t22095\tLa place\tLA\tSt. John the Baptist Parish\tH1\n70049\t22095\tEdgard\tLA\tSt. John the Baptist Parish\tH1\n70051\t22095\tGaryville\tLA\tSt. John the Baptist Parish\tH1\n71362\t22097\tPlaucheville\tLA\tSt. Landry Parish\tH1\n70584\t22097\tSunset\tLA\tSt. Landry Parish\tH1\n70525\t22097\tChurch point\tLA\tSt. Landry Parish\tH1\n70512\t22097\tArnaudville\tLA\tSt. Landry Parish\tH1\n71353\t22097\tMelville\tLA\tSt. Landry Parish\tH1\n70541\t22097\tGrand coteau\tLA\tSt. Landry Parish\tH1\n70551\t22097\tLeonville\tLA\tSt. Landry Parish\tH1\n70577\t22097\tPort barre\tLA\tSt. Landry Parish\tH1\n70550\t22097\tLawtell\tLA\tSt. Landry Parish\tH1\n70586\t22097\tVille platte\tLA\tSt. Landry Parish\tH1\n70589\t22097\tWashington\tLA\tSt. Landry Parish\tH1\n70535\t22097\tEunice\tLA\tSt. Landry Parish\tH1\n71322\t22097\tBunkie\tLA\tSt. Landry Parish\tH1\n70750\t22097\tKrotz springs\tLA\tSt. Landry Parish\tH1\n71358\t22097\tPalmetto\tLA\tSt. Landry Parish\tH1\n70571\t22097\tOpelousas\tLA\tSt. Landry Parish\tH1\n71345\t22097\tLebeau\tLA\tSt. Landry Parish\tH1\n70520\t22097\tCarencro\tLA\tSt. Landry Parish\tH1\n70570\t22097\tOpelousas\tLA\tSt. Landry Parish\tH1\n71356\t22097\tMorrow\tLA\tSt. Landry Parish\tH1\n70517\t22099\tBreaux bridge\tLA\tSt. Martin Parish\tH1\n70560\t22099\tNew iberia\tLA\tSt. Martin Parish\tH1\n70519\t22099\tCade\tLA\tSt. Martin Parish\tH1\n70380\t22099\tMorgan city\tLA\tSt. Martin Parish\tH1\n70512\t22099\tArnaudville\tLA\tSt. Martin Parish\tH1\n70563\t22099\tNew iberia\tLA\tSt. Martin Parish\tH1\n70582\t22099\tSaint martinville\tLA\tSt. Martin Parish\tH1\n70339\t22099\tPierre part\tLA\tSt. Martin Parish\tH1\n70518\t22099\tBroussard\tLA\tSt. Martin Parish\tH1\n70521\t22099\tCecilia\tLA\tSt. Martin Parish\tH1\n70540\t22101\tGarden city\tLA\tSt. Mary Parish\tH1\n70538\t22101\tFranklin\tLA\tSt. Mary Parish\tH1\n70523\t22101\tCharenton\tLA\tSt. Mary Parish\tH1\n70342\t22101\tBerwick\tLA\tSt. Mary Parish\tH1\n70380\t22101\tMorgan city\tLA\tSt. Mary Parish\tH1\n70544\t22101\tJeanerette\tLA\tSt. Mary Parish\tH1\n70522\t22101\tCenterville\tLA\tSt. Mary Parish\tH1\n70340\t22101\tAmelia\tLA\tSt. Mary Parish\tH1\n70514\t22101\tBaldwin\tLA\tSt. Mary Parish\tH1\n70392\t22101\tPatterson\tLA\tSt. Mary Parish\tH1\n70381\t22101\tMorgan city\tLA\tSt. Mary Parish\tH1\n70420\t22103\tAbita springs\tLA\tSt. Tammany Parish\tH1\n70431\t22103\tBush\tLA\tSt. Tammany Parish\tH1\n70458\t22103\tSlidell\tLA\tSt. Tammany Parish\tH1\n70433\t22103\tCovington\tLA\tSt. Tammany Parish\tH1\n70445\t22103\tLacombe\tLA\tSt. Tammany Parish\tH1\n70459\t22103\tSlidell\tLA\tSt. Tammany Parish\tH1\n70470\t22103\tMandeville\tLA\tSt. Tammany Parish\tH1\n70463\t22103\tSun\tLA\tSt. Tammany Parish\tH1\n70460\t22103\tSlidell\tLA\tSt. Tammany Parish\tH1\n70461\t22103\tSlidell\tLA\tSt. Tammany Parish\tH1\n70438\t22103\tFranklinton\tLA\tSt. Tammany Parish\tH1\n70437\t22103\tFolsom\tLA\tSt. Tammany Parish\tH1\n70452\t22103\tPearl river\tLA\tSt. Tammany Parish\tH1\n70469\t22103\tSlidell\tLA\tSt. Tammany Parish\tH1\n70427\t22103\tBogalusa\tLA\tSt. Tammany Parish\tH1\n70435\t22103\tCovington\tLA\tSt. Tammany Parish\tH1\n70448\t22103\tMandeville\tLA\tSt. Tammany Parish\tH1\n70464\t22103\tTalisheek\tLA\tSt. Tammany Parish\tH1\n70471\t22103\tMandeville\tLA\tSt. Tammany Parish\tH1\n70434\t22103\tCovington\tLA\tSt. Tammany Parish\tH1\n70447\t22103\tMadisonville\tLA\tSt. Tammany Parish\tH1\n70457\t22103\tSaint benedict\tLA\tSt. Tammany Parish\tH1\n70454\t22105\tPonchatoula\tLA\tTangipahoa Parish\tH1\n70403\t22105\tHammond\tLA\tTangipahoa Parish\tH1\n70446\t22105\tLoranger\tLA\tTangipahoa Parish\tH1\n70444\t22105\tKentwood\tLA\tTangipahoa Parish\tH1\n70466\t22105\tTickfaw\tLA\tTangipahoa Parish\tH1\n70401\t22105\tHammond\tLA\tTangipahoa Parish\tH1\n70404\t22105\tHammond\tLA\tTangipahoa Parish\tH1\n70421\t22105\tAkers\tLA\tTangipahoa Parish\tH1\n70402\t22105\tHammond\tLA\tTangipahoa Parish\tH1\n70462\t22105\tSpringfield\tLA\tTangipahoa Parish\tH1\n70451\t22105\tNatalbany\tLA\tTangipahoa Parish\tH1\n70465\t22105\tTangipahoa\tLA\tTangipahoa Parish\tH1\n70438\t22105\tFranklinton\tLA\tTangipahoa Parish\tH1\n70437\t22105\tFolsom\tLA\tTangipahoa Parish\tH1\n70436\t22105\tFluker\tLA\tTangipahoa Parish\tH1\n70442\t22105\tHusser\tLA\tTangipahoa Parish\tH1\n70422\t22105\tAmite\tLA\tTangipahoa Parish\tH1\n70443\t22105\tIndependence\tLA\tTangipahoa Parish\tH1\n70435\t22105\tCovington\tLA\tTangipahoa Parish\tH1\n70455\t22105\tRobert\tLA\tTangipahoa Parish\tH1\n70456\t22105\tRoseland\tLA\tTangipahoa Parish\tH1\n71334\t22107\tFerriday\tLA\tTensas Parish\tH1\n71357\t22107\tNewellton\tLA\tTensas Parish\tH1\n71366\t22107\tSaint joseph\tLA\tTensas Parish\tH1\n71375\t22107\tWaterproof\tLA\tTensas Parish\tH1\n71282\t22107\tTallulah\tLA\tTensas Parish\tH1\n71326\t22107\tClayton\tLA\tTensas Parish\tH1\n70360\t22109\tHouma\tLA\tTerrebonne Parish\tH1\n70343\t22109\tBourg\tLA\tTerrebonne Parish\tH1\n70364\t22109\tHouma\tLA\tTerrebonne Parish\tH1\n70344\t22109\tChauvin\tLA\tTerrebonne Parish\tH1\n70361\t22109\tHouma\tLA\tTerrebonne Parish\tH1\n70359\t22109\tGray\tLA\tTerrebonne Parish\tH1\n70352\t22109\tDonner\tLA\tTerrebonne Parish\tH1\n70301\t22109\tThibodaux\tLA\tTerrebonne Parish\tH1\n70397\t22109\tTheriot\tLA\tTerrebonne Parish\tH1\n70353\t22109\tDulac\tLA\tTerrebonne Parish\tH1\n70363\t22109\tHouma\tLA\tTerrebonne Parish\tH1\n70395\t22109\tSchriever\tLA\tTerrebonne Parish\tH1\n70377\t22109\tMontegut\tLA\tTerrebonne Parish\tH1\n70356\t22109\tGibson\tLA\tTerrebonne Parish\tH1\n71280\t22111\tSterlington\tLA\tUnion Parish\tH1\n71256\t22111\tLillie\tLA\tUnion Parish\tH1\n71260\t22111\tMarion\tLA\tUnion Parish\tH1\n71222\t22111\tBernice\tLA\tUnion Parish\tH1\n71234\t22111\tDownsville\tLA\tUnion Parish\tH1\n71241\t22111\tFarmerville\tLA\tUnion Parish\tH1\n71277\t22111\tSpearsville\tLA\tUnion Parish\tH1\n71235\t22111\tDubach\tLA\tUnion Parish\tH1\n71227\t22111\tChoudrant\tLA\tUnion Parish\tH1\n71270\t22111\tRuston\tLA\tUnion Parish\tH1\n70560\t22113\tNew iberia\tLA\tVermilion Parish\tH1\n70592\t22113\tYoungsville\tLA\tVermilion Parish\tH1\n70542\t22113\tGueydan\tLA\tVermilion Parish\tH1\n70526\t22113\tCrowley\tLA\tVermilion Parish\tH1\n70555\t22113\tMaurice\tLA\tVermilion Parish\tH1\n70575\t22113\tPerry\tLA\tVermilion Parish\tH1\n70533\t22113\tErath\tLA\tVermilion Parish\tH1\n70528\t22113\tDelcambre\tLA\tVermilion Parish\tH1\n70548\t22113\tKaplan\tLA\tVermilion Parish\tH1\n70578\t22113\tRayne\tLA\tVermilion Parish\tH1\n70529\t22113\tDuson\tLA\tVermilion Parish\tH1\n70510\t22113\tAbbeville\tLA\tVermilion Parish\tH1\n71429\t22115\tFlorien\tLA\tVernon Parish\tH1\n71438\t22115\tHineston\tLA\tVernon Parish\tH1\n71475\t22115\tSlagle\tLA\tVernon Parish\tH1\n71439\t22115\tHornbeck\tLA\tVernon Parish\tH1\n71447\t22115\tLena\tLA\tVernon Parish\tH1\n71459\t22115\tFort polk\tLA\tVernon Parish\tH1\n71474\t22115\tSimpson\tLA\tVernon Parish\tH1\n70659\t22115\tRosepine\tLA\tVernon Parish\tH1\n70634\t22115\tDeridder\tLA\tVernon Parish\tH1\n71403\t22115\tAnacoco\tLA\tVernon Parish\tH1\n71461\t22115\tNew llano\tLA\tVernon Parish\tH1\n70656\t22115\tPitkin\tLA\tVernon Parish\tH1\n71446\t22115\tLeesville\tLA\tVernon Parish\tH1\n71496\t22115\tLeesville\tLA\tVernon Parish\tH1\n71443\t22115\tKurthwood\tLA\tVernon Parish\tH1\n70639\t22115\tEvans\tLA\tVernon Parish\tH1\n70444\t22117\tKentwood\tLA\tWashington Parish\tH1\n70426\t22117\tAngie\tLA\tWashington Parish\tH1\n70438\t22117\tFranklinton\tLA\tWashington Parish\tH1\n70450\t22117\tMount hermon\tLA\tWashington Parish\tH1\n70427\t22117\tBogalusa\tLA\tWashington Parish\tH1\n70435\t22117\tCovington\tLA\t
